vi "CSM Duplicate Name Error.vi"(8 "error in (no error)":errorcluster, 10 "Occured":bool=TRUE, 11 "CSM Name":string) -> (0 "error out":errorcluster)   [LabVIEW 2017, in "Communicable State Machine.lvlib"]
uses:
  Communicable State Machine.lvlib
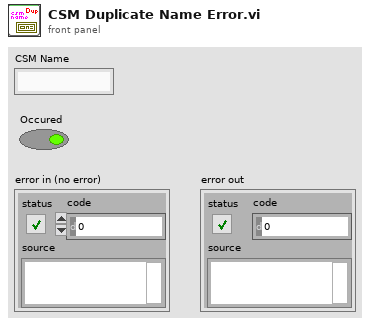
[diagram p1: front panel]
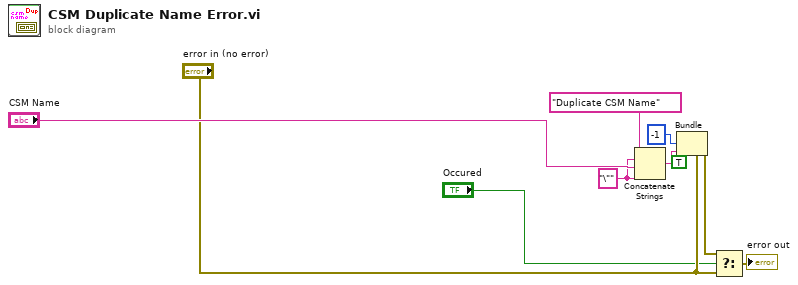
[diagram p0: block diagram]
diagram:
  w7 = "\"" ("string")
  n1 = Concatenate Strings("Duplicate CSM Name" ("String to Prepend to source (\"\")"), w7, "CSM Name", w7) -> (w6:string)
  n2 = Bundle(cluster="error in (no error)", "status"=TRUE, "code"=-1, "source"=w6) -> (w2:errorcluster)
  n3 = Select(t=w2, s="Occured", f="error in (no error)") -> (s? t:f=→"error out":errorcluster)
